vi "Button and Indicator Sizes.vi"(11 "error in (no error)":errorcluster) -> (4 "Button Width":dbl, 6 "Button Height":dbl, 8 "Numerice Indicator Width":dbl, 10 "Numeric Indicator Height":dbl, 15 "error out":errorcluster)   [LabVIEW 2014]
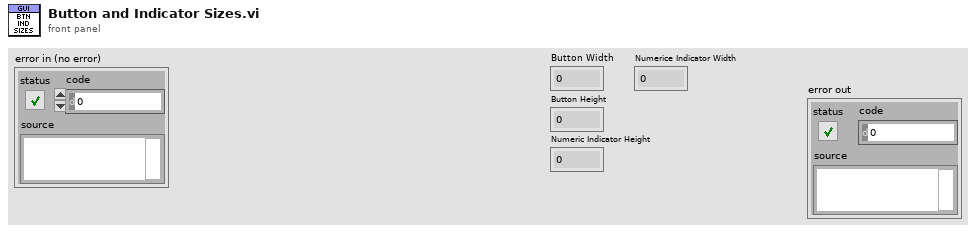
[diagram p1: front panel]
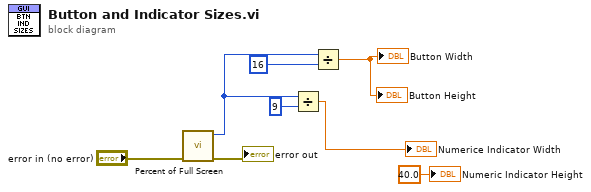
[diagram p0: block diagram]
diagram:
  n1 = call "Percent of Full Screen.vi"("error in (no error)"="error in (no error)") -> ("error out"=→"error out":errorcluster, "Right"=w4:i16)  [unwired: 8 in, 1 out]
  n2 = Divide(x=w4, y=i16 9) -> (x/y=→"Numerice Indicator Width":dbl)
  n3 = Divide(x=w4, y=16) -> (x/y=→"Button Width" →"Button Height":dbl)
  "Numeric Indicator Height" <- 40.0 ("Numeric Indicator Height")
